vi "计时器.vi"() -> (1 "时间标识":timestamp)   [LabVIEW 2016, in "TCP文件传输系统.lvlib" / "TCP接收文件.lvlib"]
panel:
  in  "停止":bool
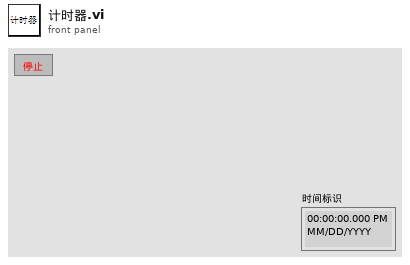
[diagram p1: front panel]
types:
  T1 = typedef "LVDateTimeRec.ctl" = cluster{"秒数的小数部分":dbl, "秒":i32, "分":i32, "时":i32, "日":i32, "月":i32, "年":i32, "天数（周）":i32, "天数（年）":i32, "DST":i32}
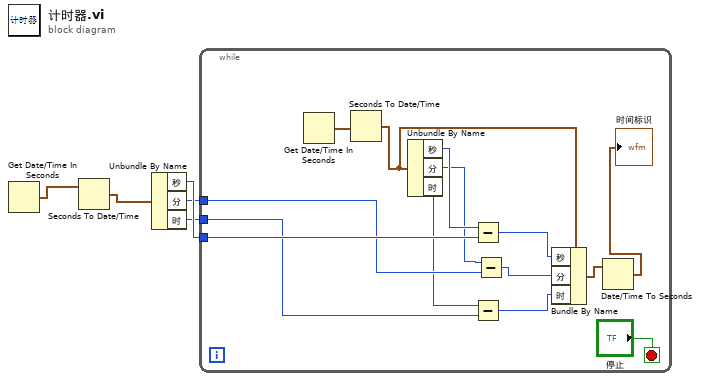
[diagram p0: block diagram]
diagram:
  n1 = Get Date/Time In Seconds() -> (seconds since 1Jan1904=w5:timestamp)
  n2 = Seconds To Date/Time(time stamp (now)=w5) -> (date time rec=w4:T1)  [unwired: 1 in]
  n3 = Unbundle By Name(w4) -> ("秒"=w3:i32, "分"=w2:i32, "时"=w1:i32)
  n4 = while {
    tunnel: w3 -> [w19]
    tunnel: w2 -> [w18]
    tunnel: w1 -> [w17]
    stop <- "停止" stop-if-true
    n5 = Get Date/Time In Seconds() -> (seconds since 1Jan1904=w16:timestamp)
    n6 = Seconds To Date/Time(time stamp (now)=w16) -> (date time rec=w9:T1)  [unwired: 1 in]
    n7 = Unbundle By Name(w9) -> ("秒"=w15:i32, "分"=w14:i32, "时"=w13:i32)
    n8 = Subtract(x=w15, y=w19) -> (x-y=w12:i32)
    n9 = Subtract(x=w13, y=w17) -> (x-y=w10:i32)
    n10 = Subtract(x=w14, y=w18) -> (x-y=w11:i32)
    n11 = Bundle By Name(cluster=w9, "秒"=w12, "分"=w11, "时"=w10) -> (w8:T1)
    n12 = Date/Time To Seconds(2:w8) -> (0:→"时间标识":timestamp)  [unwired: 1 in]
  }
